vi "Shoot-Auto.vi"(11 "Output":dbl) -> ()   [LabVIEW 2019]
uses:
  <vilib>/Rock Robotics/WPI/ThirdParty/Phoenix-LabVIEW/Motor Controller/Controls/CTRE_Phoenix_MotorControl_ControlMode.ctl
  Robot Global Data.vi
  <vilib>/Rock Robotics/WPI/ThirdParty/Phoenix-LabVIEW/Motor Controller/Get/CTRE_Phoenix_MotorController_IntegratedSensorData_TalonFX.vi
panel:
  out "Run":bool
  in  "Output 2":dbl=-4000.0
  out "WVelocity":dbl
  out "MVelocity":dbl
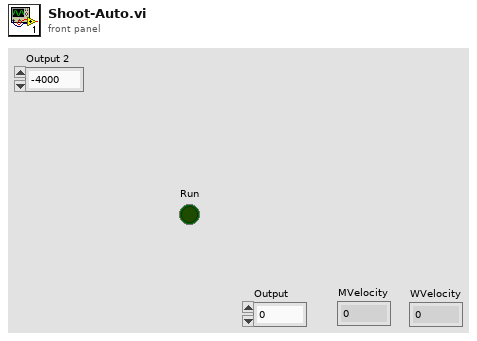
[diagram p1: front panel]
types:
  T1 = typedef "CTRE_Phoenix_MotorControl_ControlMode.ctl" = u16
  T2 = typedef "WPI_MotorControlDeviceRef.ctl" = cluster{"DeviceStatus":errorcluster, "Type":T3, "PWM":cluster{"PWM Channel":T4, "DeadBand":T5}, "CAN":cluster{"Device Number":u8, "SetOutput VI Ref":variant, "GetOutput VI Ref":variant, "Enable VI Ref":variant, "Disable VI Ref":variant, "Data":variant}, "Invert":bool, "DIO PWM":cluster{"PWM \"Enable\" Channel":T4, "DIOChannel":T6, "PWM Rate":dbl}}
  T3 = typedef "WPI_MotorControlType.ctl" = enum16{"PWM", "CAN", "DIO PWM"}
  T4 = typedef "FPGA_DIOPWMChannel.ctl" = enum8{"PWM 0", "PWM 1", "PWM 2", "PWM 3", "PWM 4", "PWM 5", "PWM 6", "PWM 7", "PWM 8", "PWM 9", "PWM MXP 0", "PWM MXP 1", "PWM MXP 2", "PWM MXP 3", "PWM MXP 4", "PWM MXP 5", "PWM MXP 6", "PWM MXP 7", "PWM MXP 8", "PWM MXP 9", "Invalid"}
  T5 = typedef "WPI_PWMDeadband.ctl" = cluster{"Name":string, "maxPositivePwm":i32, "minPositivePwm":i32, "centerPwm":i32, "maxNegativePwm":i32, "minNegativePwm":i32, "angularRange":u16}
  T6 = typedef "FPGA_DIOChannel.ctl" = enum8{"DIO 0", "DIO 1", "DIO 2", "DIO 3", "DIO 4", "DIO 5", "DIO 6", "DIO 7", "DIO 8", "DIO 9", "DIO MXP 0", "DIO MXP 1", "DIO MXP 2", "DIO MXP 3", "DIO MXP 4", "DIO MXP 5", "DIO MXP 6", "DIO MXP 7", "DIO MXP 8", "DIO MXP 9", "DIO MXP 10", "DIO MXP 11", "DIO MXP 12", "DIO MXP 13", "DIO MXP 14", "DIO MXP 15", "SPI Port CS1", "SPI Port CS2", "SPI Port CS3", "SPI Port MISO", "SPI Port MOSI", "Invalid"}
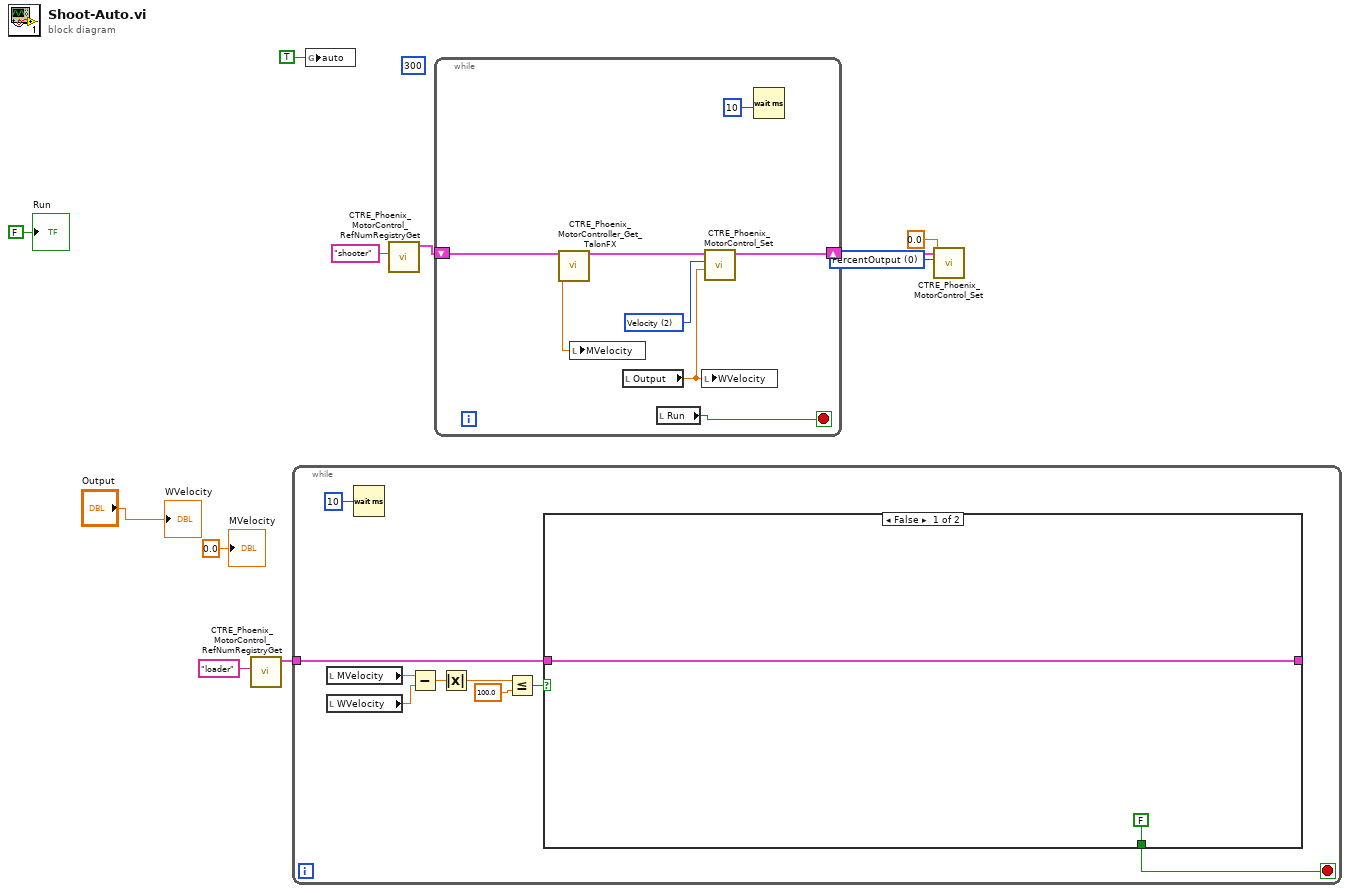
[diagram p0: block diagram]
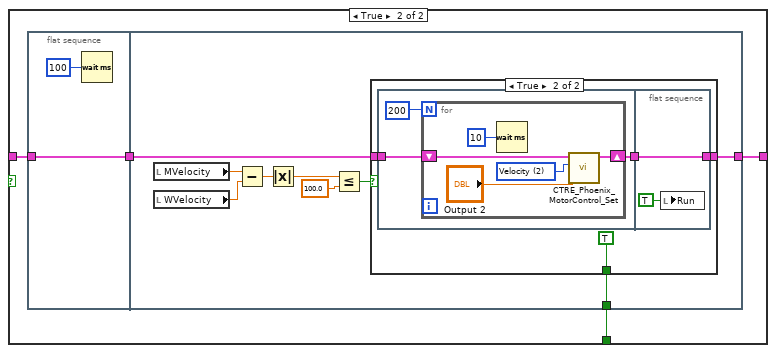
[diagram p2: hidden frame]
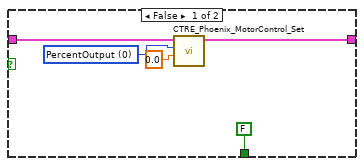
[diagram p3: hidden frame]
diagram:
  w2 = T1 0 items=["PercentOutput"=0, "Position"=1, "Velocity"=2, "Current"=3, "Follower"=5, "MotionProfile"=6, "MotionMagic"=7, "MotionProfileArc"=10, "Disabled"=15] ("Control Mode")
  (unwired) 300
  n1 = call <vilib>:"CTRE_Phoenix_MotorControl_RefNumRegistryGet.vi"("refnum name"="loader") -> ("PhoenixMotorControlDevRef"=w9:T2)  [unwired: 9 in, 1 out]
  n2 = while {
    tunnel: w9 -> [w14]
    stop <- w12 stop-if-true
    n3 = local read "MVelocity"() -> (w18:dbl)
    n4 = local read "WVelocity"() -> (w17:dbl)
    n5 = Wait (ms)(milliseconds to wait=u32 10) -> ()  [unwired: 1 out]
    n6 = Subtract(x=w18, y=w17) -> (x-y=w19:dbl)
    n7 = Absolute Value(x=w19) -> (abs(x)=w20:dbl)
    n8 = Less Or Equal?(x=w20, y=100.0) -> (x <= y?=w15:bool)
    n9 = case shown="False" w15 {
      tunnel: [w22 w26] -> _
      tunnel: w14 -> [w22 w24]
      tunnel: [FALSE w23] -> w12
      frame False {
      }
      frame True {
        n10 = flat-sequence {
          tunnel: w24 -> [w27]
          tunnel: [w27] -> w25
          tunnel: [w31] -> w26
          tunnel: w25 -> [w30]
          tunnel: [w29] -> w23
          frame #0 {
            n11 = Wait (ms)(milliseconds to wait=u32 100) -> ()  [unwired: 1 out]
          }
          frame #1 {
            n12 = local read "MVelocity"() -> (w34:dbl)
            n13 = local read "WVelocity"() -> (w33:dbl)
            n14 = Subtract(x=w34, y=w33) -> (x-y=w36:dbl)
            n15 = Absolute Value(x=w36) -> (abs(x)=w37:dbl)
            n16 = Less Or Equal?(x=w37, y=100.0) -> (x <= y?=w32:bool)
            n17 = case shown="True" w32 {
              tunnel: [w40 w46] -> w31
              tunnel: w30 -> [w39 w45]
              tunnel: [FALSE TRUE] -> w29
              frame False {
                w42 = T1 0 items=["PercentOutput"=0, "Position"=1, "Velocity"=2, "Current"=3, "Follower"=5, "MotionProfile"=6, "MotionMagic"=7, "MotionProfileArc"=10, "Disabled"=15] ("Control Mode")
                n18 = call <vilib>:"CTRE_Phoenix_MotorControl_Set.vi"("Output"=0.0, "Control Mode"=w42, "PhoenixMotorControlDevRef"=w39) -> ("PhoenixMotorControlDevRef"=w40:T2)  [unwired: 7 in, 1 out]
              }
              frame True {
                n19 = flat-sequence {
                  tunnel: w45 -> [w47]
                  tunnel: [w49] -> w43
                  tunnel: [w56] -> w46
                  tunnel: w43 -> [w56]
                  frame #0 {
                    n20 = for {
                      N: 200 -> [_]
                      shift-right: [w53] -> w49
                      shift-left: w47 -> [w54]
                      w52 = T1 2 items=["PercentOutput"=0, "Position"=1, "Velocity"=2, "Current"=3, "Follower"=5, "MotionProfile"=6, "MotionMagic"=7, "MotionProfileArc"=10, "Disabled"=15] ("Control Mode")
                      n21 = Wait (ms)(milliseconds to wait=u32 10) -> ()  [unwired: 1 out]
                      n22 = call <vilib>:"CTRE_Phoenix_MotorControl_Set.vi"("Output"="Output 2", "Control Mode"=w52, "PhoenixMotorControlDevRef"=w54) -> ("PhoenixMotorControlDevRef"=w53:T2)  [unwired: 7 in, 1 out]
                    }
                  }
                  frame #1 {
                    n23 = local write "Run"(TRUE ("Run")) -> ()
                  }
                }
              }
            }
          }
        }
      }
    }
  }
  n24 = global write "Robot Global Data.vi" "auto"(TRUE ("auto")) -> ()
  n25 = call <vilib>:"CTRE_Phoenix_MotorControl_RefNumRegistryGet.vi"("refnum name"="shooter") -> ("PhoenixMotorControlDevRef"=w7:T2)  [unwired: 9 in, 1 out]
  n26 = while {
    shift-right: [w59] -> w3
    shift-left: w7 -> [w64]
    stop <- w57 stop-if-true
    w61 = T1 2 items=["PercentOutput"=0, "Position"=1, "Velocity"=2, "Current"=3, "Follower"=5, "MotionProfile"=6, "MotionMagic"=7, "MotionProfileArc"=10, "Disabled"=15] ("Control Mode")
    n27 = call-poly <vilib>:"CTRE_Phoenix_MotorController_Get_TalonFX.vi"("PhoenixMotorControlDevRef"=w64) -> ("PhoenixMotorControlDevRef"=w63:T2, "Velocity"=w62:dbl)  [unwired: 10 in, 3 out]
    n28 = local write "MVelocity"(w62) -> ()
    n29 = local read "Output"() -> (w60:dbl)
    n30 = local read "Run"() -> (w57:bool)
    n31 = local write "WVelocity"(w60) -> ()
    n32 = call <vilib>:"CTRE_Phoenix_MotorControl_Set.vi"("Output"=w60, "Control Mode"=w61, "PhoenixMotorControlDevRef"=w63) -> ("PhoenixMotorControlDevRef"=w59:T2)  [unwired: 7 in, 1 out]
    n33 = Wait (ms)(milliseconds to wait=u32 10) -> ()  [unwired: 1 out]
  }
  n34 = call <vilib>:"CTRE_Phoenix_MotorControl_Set.vi"("Output"=0.0, "Control Mode"=w2, "PhoenixMotorControlDevRef"=w3) -> ()  [unwired: 7 in, 2 out]
  "MVelocity" <- 0.0 ("MVelocity")
  "WVelocity" <- "Output"
  "Run" <- FALSE ("Run")
